vi "play-batch-raster-scan.vi"() -> ()   [LabVIEW 2017]
uses:
  raster-scan-params.ctl
  controls/PI-params.ctl
  controls/boolean_info.ctl
  controls/raster_input_meta_data.ctl
  <vilib>/userdefined/High Color/nirio_resource_hc.ctl
  controls/rasterMetaData.ctl
  <vilib>/FPGAPlugInAG/cRIO-9082/niLvFpga_Open_cRIO-9082.vi
  <vilib>/rvi/interface/common/dynamic/niFpgaDynamicAddResources.vi
  <vilib>/FPGAPlugInAG/Dynamic/niLvFpga_Reset_Dynamic.vi
  <vilib>/rvi/interface/common/niFpgaWaitOnOcc.vi
  <vilib>/Utility/error.llb/Error Cluster From Error Code.vi
  <vilib>/rvi/errors/niLvFpgaAdjustHostInterfaceError.vi
  <vilib>/FPGAPlugInAG/Dynamic/niLvFpga_Run_Dynamic.vi
  <vilib>/Utility/file.llb/Read Delimited Spreadsheet (DBL).vi
  <vilib>/FPGAPlugInAG/Dynamic/niLvFpga_Close_Dynamic.vi
  <userlib>/_matio/level5/Public/Write/Append Data Element.llb/Append Data Element (Anything).vi
  <vilib>/rvi/interface/nirviOpenFPGA/nirviOpenFPGA.xnode
  FPGA Bitfiles/afmimagingcontro_FPGATargetSPARTA_raster-scanning_DXF4O8EAjZ4.lvbitx
  <vilib>/rvi/interface/nirviMethod/nirviMethod.xnode
  <vilib>/rvi/interface/nirviReadWriteControl/nirviReadWriteControl.xnode
  <vilib>/rvi/interface/nirviCloseFPGA/nirviCloseFPGA.xnode
  <vilib>/FPGAPlugInAG/Dynamic/niLvFpga_ConfigureFifo_Dynamic.vi
  <vilib>/rvi/errors/niLvFpgaMergeErrorWithErrorCode.vi
  <vilib>/rvi/interface/Simulation/niFpgaSimulationCallBeginRW.vi
  <vilib>/FPGAPlugInAG/Dynamic/niLvFpga_ReadFifo_Dynamic.vi
  NiFpgaLv.dll
  <userlib>/_matio/level5.lvlib
  <vilib>/FPGAPlugInAG/Dynamic/niLvFpga_WriteFifo_Dynamic.vi
panel:
  out "Array 2":path[](array[path])
  out "control":dbl[](graph)
  out "error":dbl[](graph)
  out "InputMetaData":T1
  out "output-meta-data-path":path
  in  "Tab Control":enum32{"Page 1", "Debug"}(tab)
  in  "data-root":path=path "C:/Users/arnold/Documents/labview/afm_imaging/data/raster/5microns"
  in  "number-of-pixels":i32=256
  out "points_per_line":i32=250000
  out "total_num_points":i32
  in  "raise-constant (init)":sgl
  in  "raise-constant":sgl
  in  "trigger-0":bool
  in  "STOP":bool
  in  "xy-init":fxp<+/-,16,5>[](array[numeric])=[0.0, 0.0]
  in  "Ki-xy":dbl=0.01 format="%#_13g"
  out "ADC-zaxis":sgl
  out "DAC-zaxis":sgl
  in  "xy-bound":sgl=7.0
  out "current_output-data-path":path
  in  "note-blob":string
  in  "overwrite":bool
  in  "raster-scan-params":T2={"TsTicks"=1600, "Stop"=FALSE, "TOL"=0.3, "ramp-rate"=-5e-05, "z-u-max"=5.0, "PI-params"={"Ki"=0.01, "setpoint"=0.0}, "Num"=[1.0, 0.0, 0.0, 0.0, 0.0, 0.0, 0.0, 0.0, 0.0], "TF Order"=1, "Den"=[1.0, 0.0, 0.0, 0.0, 0.0, 0.0, 0.0, 0.0, 0.0]} {"ramp-rate" format="%#_5g"; "TOL" format="%#_13g"}
  in  "do-Dz":bool
  in  "do_xy_CL":bool
  out "boolean errors":T4
  in  "Z-settle-N":i16=10000
  in  "Array":string[](array[string])
  out "Actual Depth":u32
  out "Elements Remaining":u32
  out "size(s)":i32
  out "y iter":i32
  out "nsamps 2":i32
  out "Empty Elements Remaining":u32
  out "(int) y*floor(x/y)":u64
  out "elements left 2":i32=1
  out "x >= y?":bool
  out "writing stopped":bool
  out "size(s) 2":i32
  out "case-selector-feedback":i16
  out "e(0) (threshhold init)":fxp<+/-,16,5>
  out "total-time":dbl
  out "x+1":i32
  out "que timed out?":bool
  out "Error signal (previous line) 2":dbl[](graph)
  out "Waveform Graph":dbl[](graph)
  out "base y_ref (ramp)":dbl[](graph)
  out "base x_ref(triangle wave)":dbl[](graph)
  out "Intensity Graph":dbl[][](graph)
  out "Error signal (previous line)":dbl[](graph)
  # "x-axis"
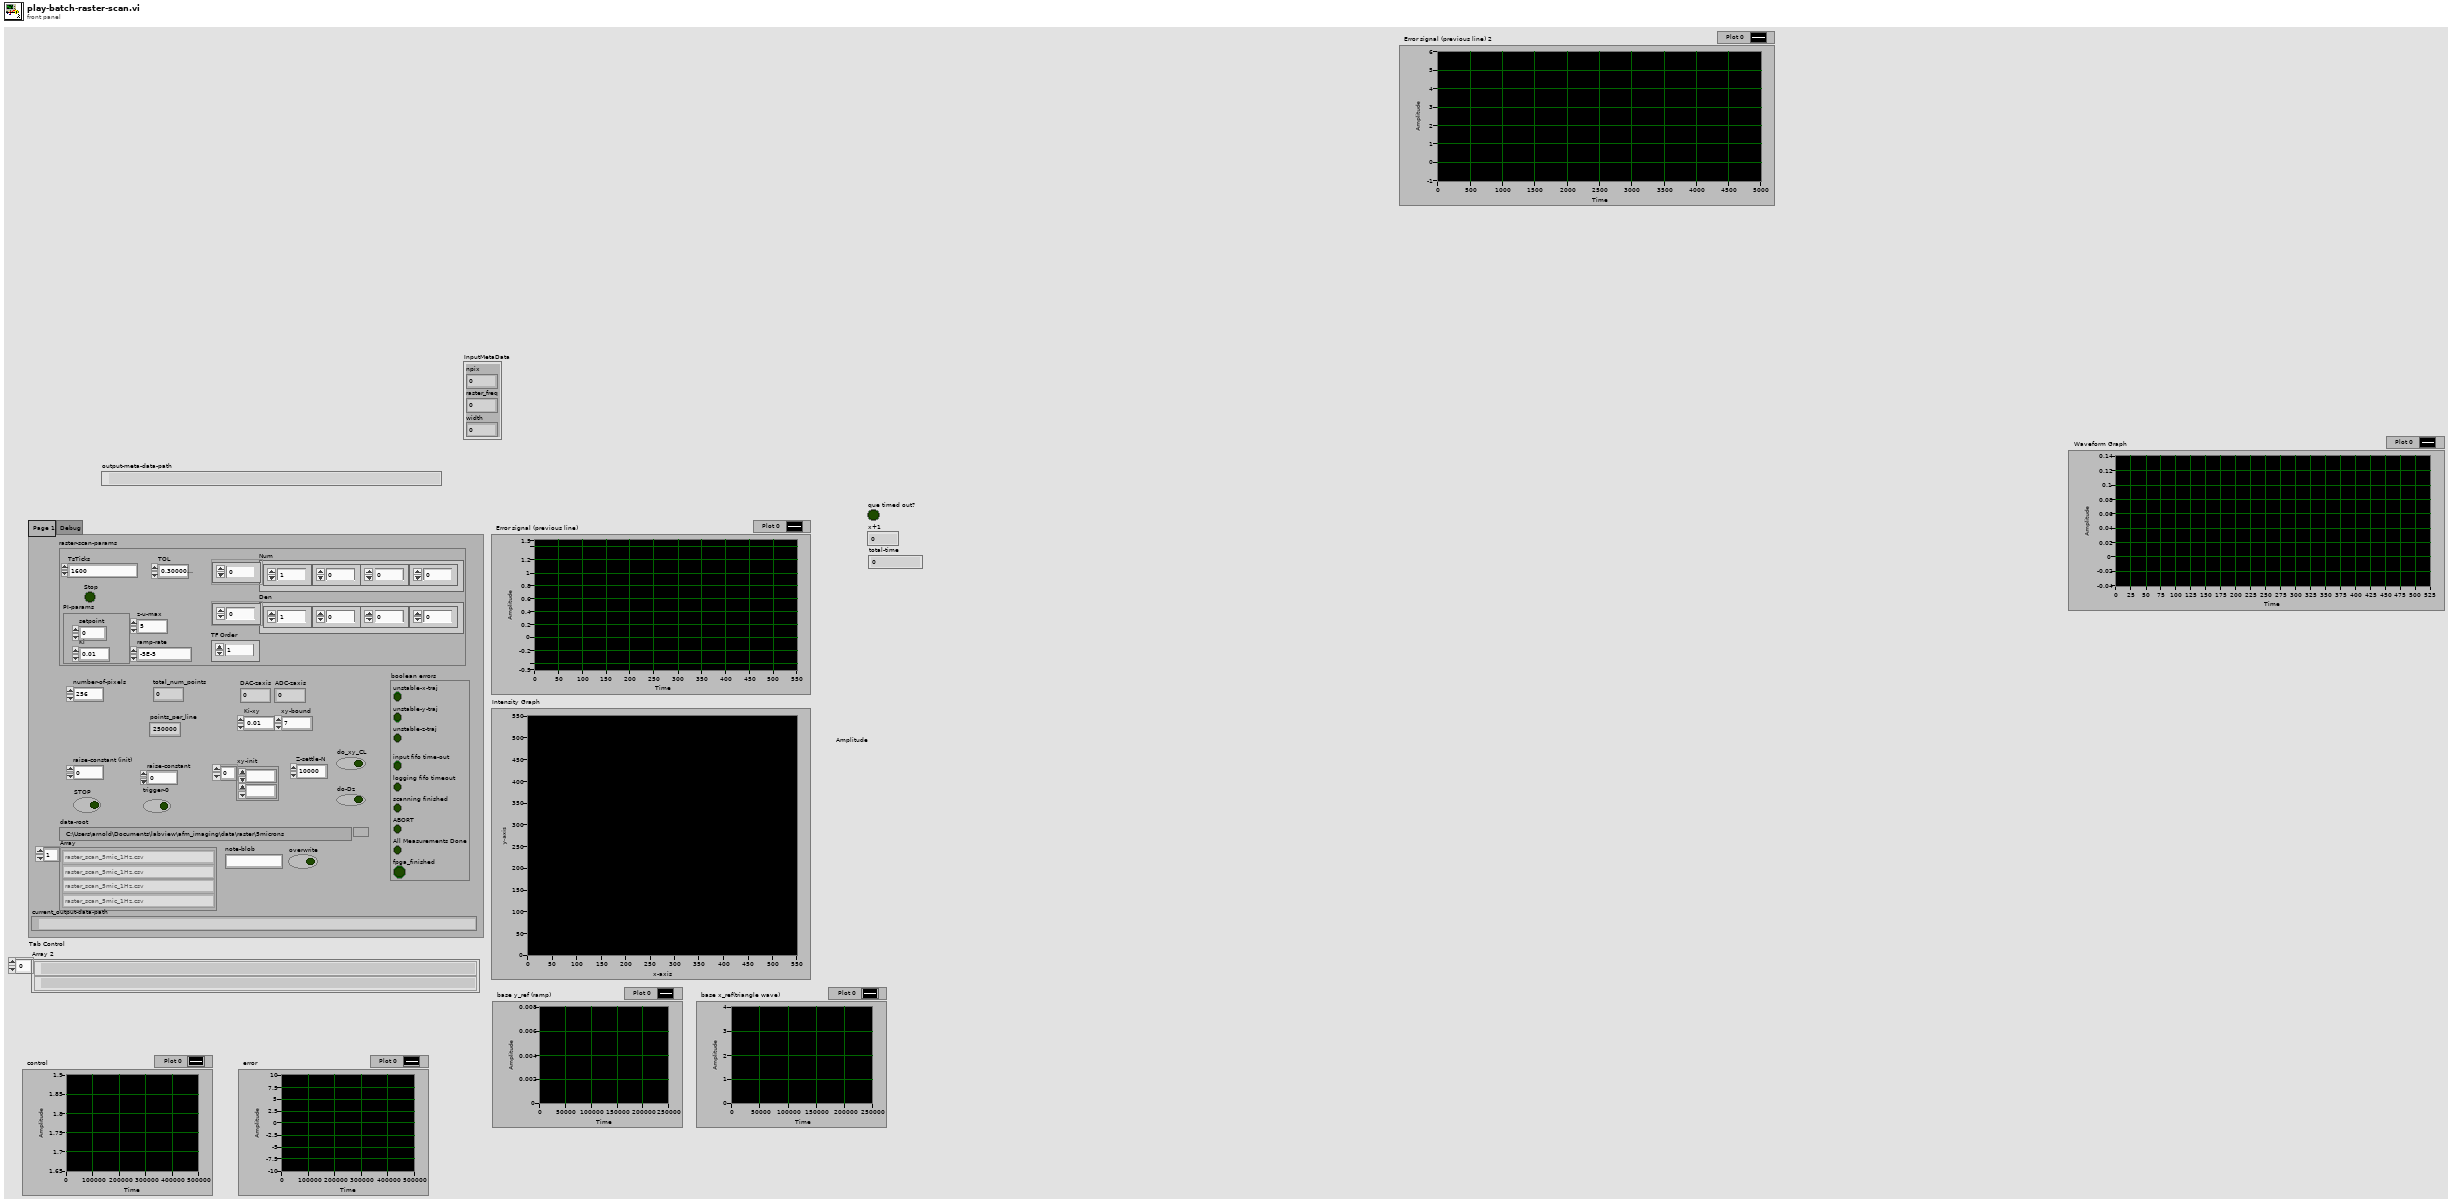
[diagram p1: front panel]
types:
  T1 = typedef "raster_input_meta_data.ctl" = cluster{"npix":dbl, "raster_freq":dbl, "width":dbl}
  T2 = typedef "raster-scan-params.ctl" = cluster{"TsTicks":u32, "Stop":bool, "TOL":sgl, "ramp-rate":sgl, "z-u-max":sgl, "PI-params":T3, "Num":sgl[], "TF Order":i32, "Den":sgl[]}
  T3 = typedef "PI-params.ctl" = cluster{"Ki":sgl, "setpoint":sgl}
  T4 = typedef "boolean_info.ctl" = cluster{"unstable-z-traj":bool, "input fifo time-out":bool, "logging fifo timeout":bool, "scanning finished":bool, "unstable-x-traj":bool, "unstable-y-traj":bool, "ABORT":bool, "All Measurements Done":bool, "fpga_finished":bool}
  T5 = typedef "nirio_resource_hc.ctl" = tag
  T6 = typedef "rasterMetaData.ctl" = cluster{"raster-scan-params":T2, "xy-bound":sgl, "DAC-zaxis":sgl, "ADC-zaxis":sgl, "Ki-xy":dbl, "total_num_points":i32, "points_per_line":i32, "number-of-lines":i32, "number-of-pixels":i32, "raster_meta_in":T1}
  T7 = enum16{"open", "replace", "create", "open or create", "replace or create", "replace or create with confirmation"}
  T8 = cluster{"unstable-z-traj":bool, "input fifo time-out":bool, "logging fifo timeout":bool, "scanning finished":bool, "unstable-x-traj":bool, "unstable-y-traj":bool, "ABORT":bool, "All Measurements Done":bool, "fpga_finished":bool}
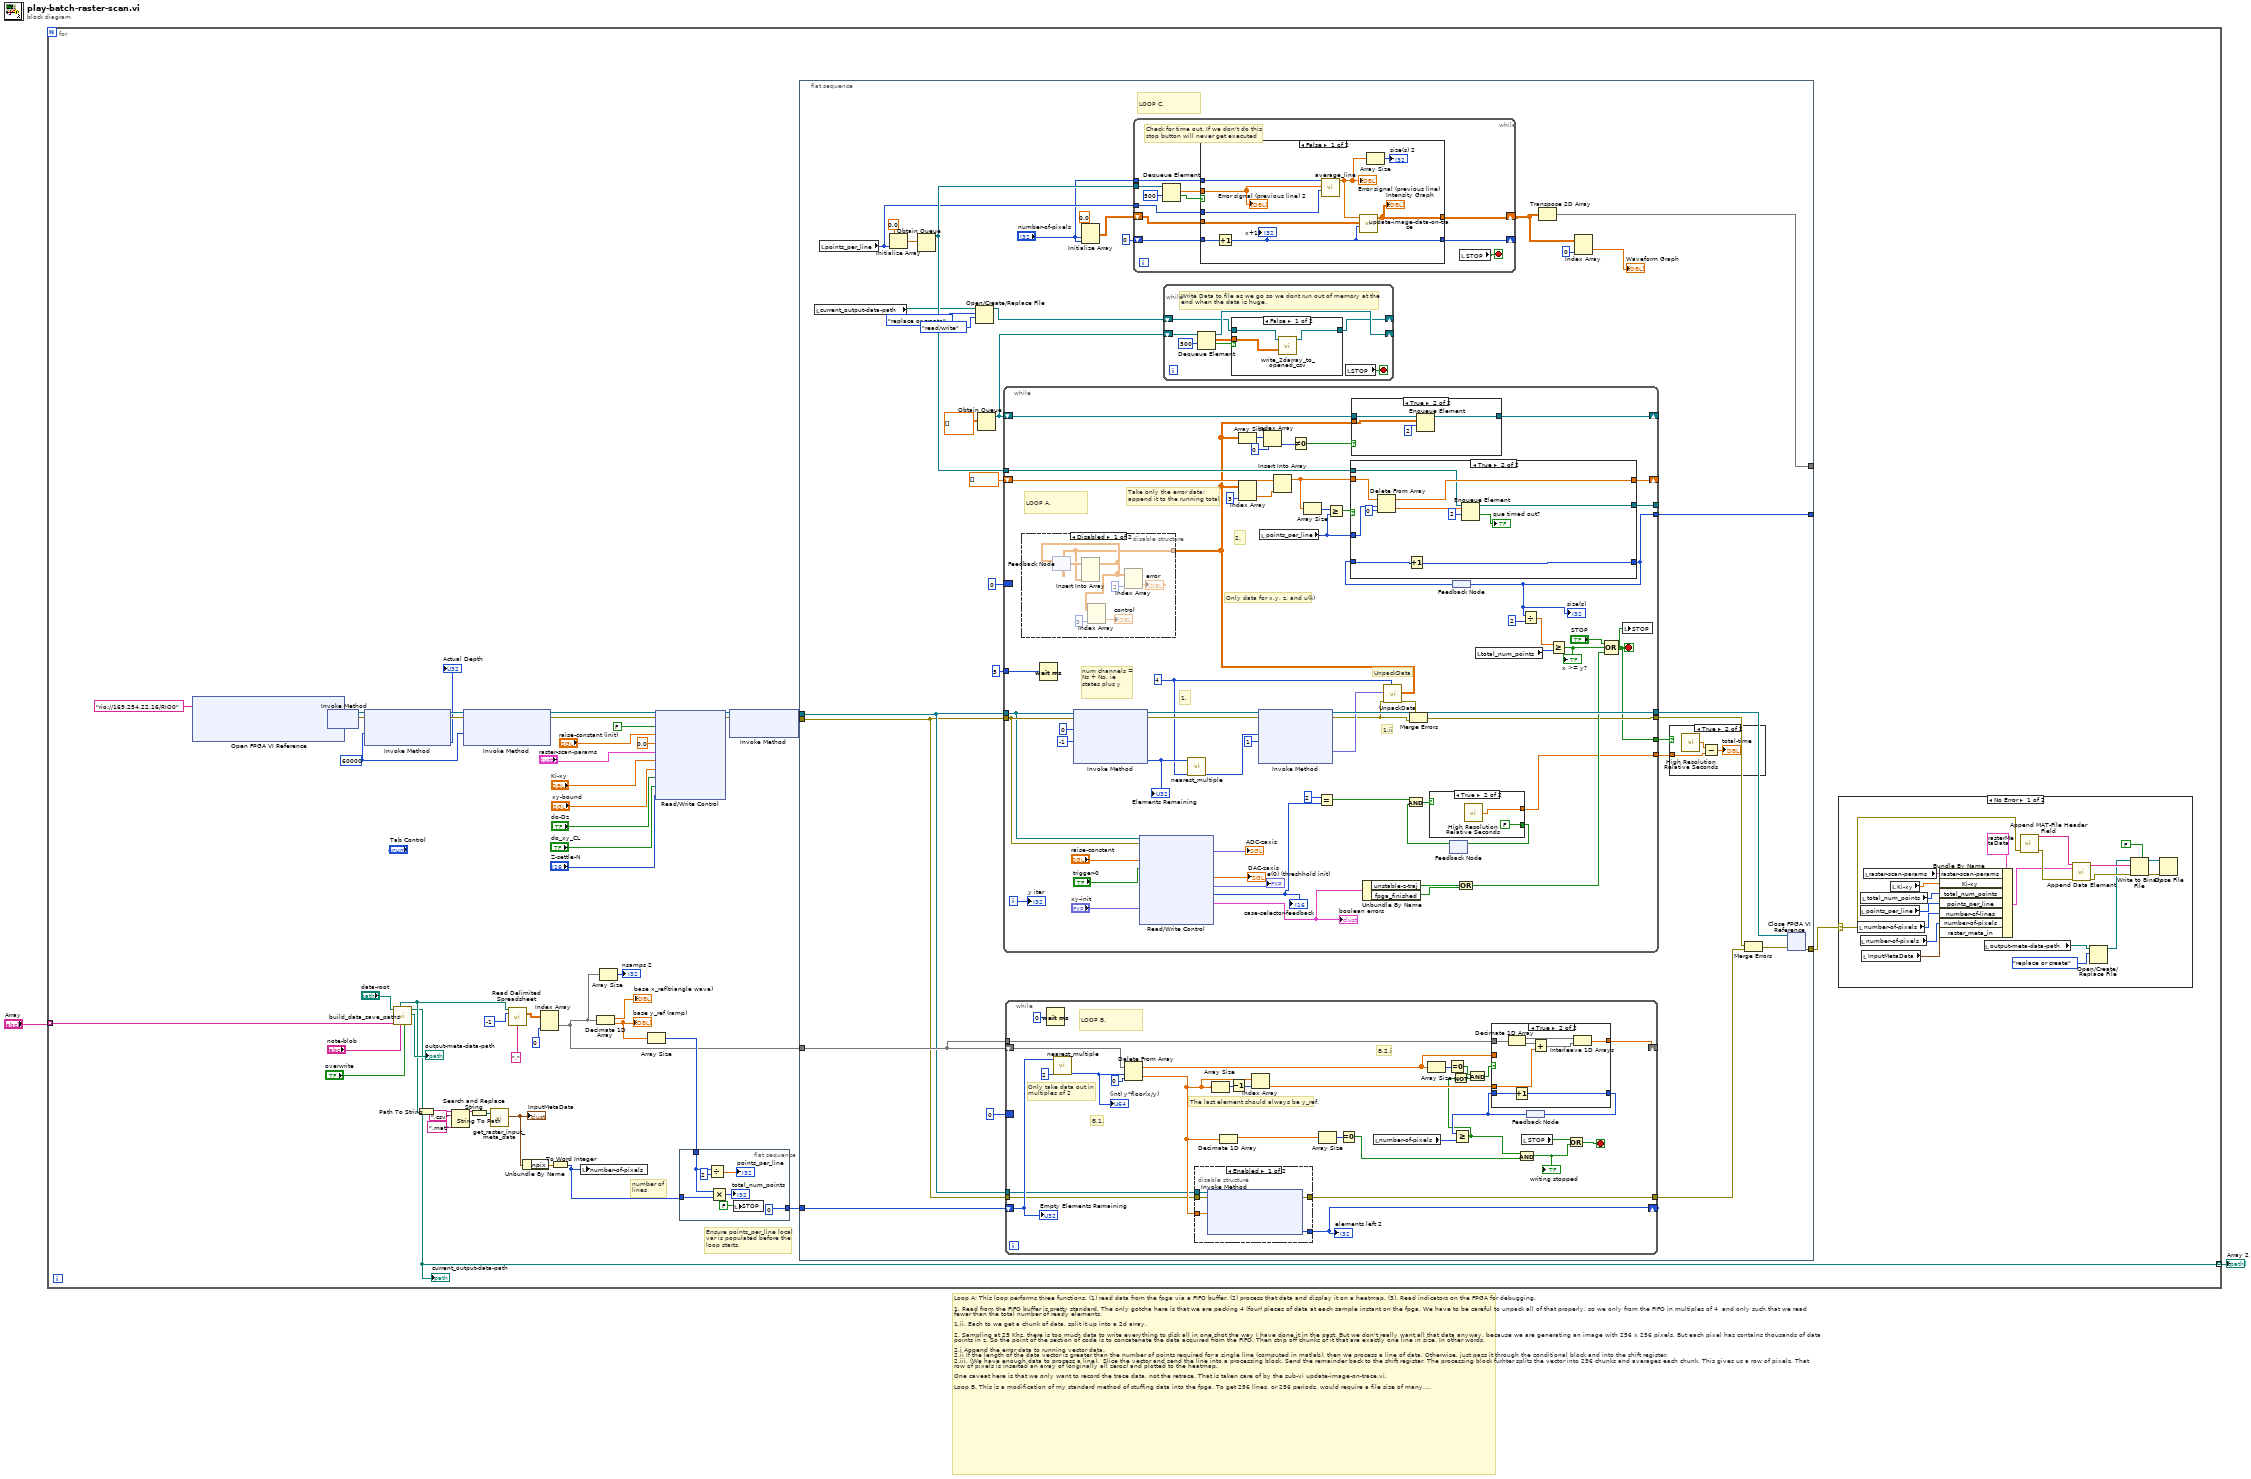
[diagram p0: block diagram]
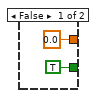
[diagram p8: hidden frame]
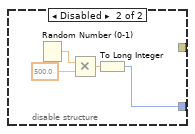
[diagram p11: hidden frame]
diagram:
  # "Loop A; This loop performs three functions. (1) read data from the fpga via a FIFO buffer. (2) process that data and display it on a heatmap. (3). Read indicators on the FPGA for debugging.\n\n1. Read from the FIFO buffer is pretty standard. The only gotcha here is that we are packing 4 (four) pieces of data at each sample instant on the fpga. We have to be careful to unpack all of that properly, so we only from the FIFO in multiples of 4  and only such that we read fewer than the total number of ready elements. \n\n1.ii. Each to we get a chunk of data, split it up into a 2d array. \n\n2. Sampling at 25 Khz, there is too much data to write everything to disk all in one shot the way I have done it in the past. But we don't really want all that data anyway, because we are generating an image with 256 x 256 pixels. But each pixel has contains thousands of data points in z. So the point of the section of code is to concatenate the data acquired from the FIFO. Then strip off chunks of it that are exactly one line in size. In other words,\n\n2.i Append the error data to running vector data.\n2.ii If the length of the data vector is greater than the number of points required for a single line (computed in matlab), then we process a line of data. Otherwise, just pass it through the conditional block and into the shift register. \n2.iii. (We have enough data to process a line).  Slice the vector and send the line into a processing block. Send the remainder back to the shift register. The processing block furhter splits the vector into 256 chunks and averages each chunk. This gives us a row of pixels. That row of pixels is inserted an array of (originally all zeros) and plotted to the heatmap.\n\nOne caveat here is that we only want to record the trace data, not the retrace. That is taken care of by the sub-vi update-image-on-trace.vi.\n\nLoop B. This is a modification of my standard method of stuffing data into the fpga. To get 256 lines, or 256 periods, would require a file size of many, many gigibtyes. SO the point here is to only use a single period of the triangle wave and corresponding ramp signal. Everytime we exauhst that data, re-cycle the same data and keep pumping it back in. The one tricky part here is that we have to be careful to shift the original ramp data up by the appropriate amount. We also have to take special care because of how the data is packed from matlab. [x(1), y(1), x(2), y(2)...].\n\nThe first iteration of the loop, we don't push any data in. All we do is get the number of empty elements.\n\nB.1 Each iteration, strip off ' empty elements ' elements from the array and send them to FIFO. \nB.2.i Is the remaining array empty?\nB.2.ii Grab the very last element. We need this"
  n1 = for {
    tunnel: "Array" -> [w4] mode=indexing
    tunnel: [w3] -> w1 mode=indexing
    w50 = 60000
    # "number of \nlines"
    # "Ensure points_per_line local\nvar is populated before the\nloop starts."
    n2 = xnode "Open FPGA VI Reference"("resource name"=T5 "rio://169.254.22.16/RIO0") -> ("FPGA VI Reference Out"=w49:refnum<k20>, "error out"=w48:errorcluster)  [unwired: 1 in]
    n3 = xnode "Invoke Method"("FPGA VI Reference In"=w49, "error in"=w48) -> ("FPGA VI Reference Out"=w44:refnum<k20>, "error out"=w43:errorcluster)
    n4 = xnode "Invoke Method"("FPGA VI Reference In"=w44, "error in"=w43, "Requested Depth"=w50) -> ("FPGA VI Reference Out"=w45:refnum<k20>, "error out"=w46:errorcluster, "Actual Depth"=→"Actual Depth":u32)
    n5 = call "build_data_save_paths.vi"("overwrite"="overwrite", "note-blob"="note-blob", "base-file-name"=w4, "data-root"="data-root") -> ("output-meta-data-path"=→"output-meta-data-path":path, "output-data-path"=w3:path, "input-data-path"=w13:path)  [unwired: 3 in, 2 out]
    "current_output-data-path" <- w3
    n6 = Path To String(path=w13) -> (string=w12:string)
    n7 = Search and Replace String(input string=w12, search string=".csv", replace string=".mat" ("replace string (\"\")")) -> (result string=w9:string)  [unwired: 5 in, 3 out]
    n8 = xnode "Invoke Method"("FPGA VI Reference In"=w45, "error in"=w46, "Requested Depth"=w50) -> ("FPGA VI Reference Out"=w52:refnum<k20>, "error out"=w51:errorcluster)  [unwired: 1 out]
    n9 = String To Path(string=w9) -> (path=w8:path)
    n10 = call "get_raster_input_meta_data.vi"("Path"=w8) -> ("cluster"=w7:T1)  [unwired: 10 in]
    "InputMetaData" <- w7
    n11 = call-poly <vilib>:"Read Delimited Spreadsheet.vi"("file path (dialog if empty)"=w13, "number of rows (all:-1)"=-1, "delimiter (\\t)"=",") -> ("all rows"=w30:dbl[][])  [unwired: 7 in, 5 out]
    n12 = Unbundle By Name(w7) -> ("npix"=w6:dbl)
    n13 = Index Array(array=w30, index (col)=0 ("dimension size")) -> (element=w29:dbl[])  [unwired: 1 in]
    n14 = To Word Integer(number=w6) -> (16bit integer=w5:i16)
    n15 = local write "number-of-pixels"(w5) -> ()
    n16 = Decimate 1D Array(w29) -> (→"base x_ref(triangle wave)":dbl[], w36:dbl[])
    "base y_ref (ramp)" <- w36
    n17 = Array Size(array=w29) -> (size(s)=→"nsamps 2":i32)
    n18 = Array Size(array=w36) -> (size(s)=w34:i32)
    n19 = xnode "Read/Write Control"("FPGA VI Reference In"=w52, "error in"=w51, "trigger-0"=FALSE ("constant 2 lower"), "raise-constant"="raise-constant (init)", "u(0)"=sgl 0.0, "raster-scan-params"="raster-scan-params", "Ki-xy"="Ki-xy", "xy-bound"="xy-bound", "do-Dz"="do-Dz", "do_xy_CL"="do_xy_CL", "Z-settle-N"="Z-settle-N") -> ("FPGA VI Reference Out"=w26:refnum<k20>, "error out"=w25:errorcluster)
    n20 = flat-sequence {
      tunnel: [0] -> w35
      tunnel: w34 -> [w285]
      tunnel: w5 -> [w288]
      frame #0 {
        n21 = Divide(x=w285, y=2) -> (x/y=→"points_per_line":dbl)
        n22 = Multiply(x=w285, y=w288) -> (x*y=→"total_num_points":i32)
        n23 = local write "STOP"(FALSE ("STOP")) -> ()
      }
    }
    n24 = xnode "Invoke Method"("FPGA VI Reference In"=w26, "error in"=w25) -> ("FPGA VI Reference Out"=w23:refnum<k20>, "error out"=w24:errorcluster)  [unwired: 1 in]
    n25 = flat-sequence {
      tunnel: [w82] -> _
      tunnel: w23 -> [w91]
      tunnel: w24 -> [w90]
      tunnel: w35 -> [w103]
      tunnel: w29 -> [w92]
      tunnel: [w76] -> _
      tunnel: [w73] -> w17
      frame #0 {
        # "LOOP C."
        n26 = local read "current_output-data-path"() -> (w75:path)
        n27 = local read "points_per_line"() -> (w88:i32)
        n28 = Initialize Array(0.0 ("element"), w88) -> (w97:dbl[])
        n29 = Obtain Queue(element data type=w97) -> (queue out=w94:refnum<queue>)  [unwired: 4 in, 2 out]
        n30 = Open/Create/Replace File(file path (use dialog)=w75, operation (0:open)=T7."replace or create", access (0:read/write)=enum16{"read/write", "read-only", "write-only"}."read/write") -> (refnum out=w77:refnum<file>)  [unwired: 3 in, 2 out]
        n31 = Obtain Queue(element data type=dbl[][] []) -> (queue out=w80:refnum<queue>)  [unwired: 4 in, 2 out]
        n32 = while {
          tunnel: 5 -> [w202]
          tunnel: w91 -> [w193]
          tunnel: w90 -> [w194]
          tunnel: [w173] -> w85
          tunnel: [w196] -> w86
          shift-right: [w185] -> _
          shift-left: dbl[] [] -> [w183]
          border: 0 ("disabled index (col)") -> [_]
          tunnel: w94 -> [w164]
          tunnel: [w163] -> _
          tunnel: [w161] -> w84
          tunnel: [w154] -> w83
          shift-right: [w148] -> _
          shift-left: w80 -> [w147]
          tunnel: [w146] -> w76
          i -> [w192]
          stop <- w161 stop-if-true
          w170 = u32 4 ("y")
          # "2."
          # "1.ii"
          # "1."
          # "LOOP A."
          # "Take only the error data;\nappend it to the running total"
          # "num channels = Ns + No, ie states plus y"
          # "Only data for x,y, z, and u(k)"
          # "UnpackData"
          n33 = Wait (ms)(milliseconds to wait=w202) -> ()  [unwired: 1 out]
          n34 = xnode "Invoke Method"("FPGA VI Reference In"=w193, "error in"=w194, "Number of Elements"=0 ("Timeout (ms)"), "Timeout (ms)"=-1) -> ("FPGA VI Reference Out"=w198:refnum<k20>, "error out"=w199:errorcluster, "Elements Remaining"=w171:u32)  [unwired: 1 out]
          "Elements Remaining" <- w171
          n35 = xnode "Read/Write Control"("FPGA VI Reference In"=w193, "error in"=w194, "raise-constant"="raise-constant", "trigger-0"="trigger-0", "xy-init"="xy-init") -> ("ADC-zaxis"=→"ADC-zaxis":fxp<+/-,24,5>, "DAC-zaxis"=→"DAC-zaxis":sgl, "e(0) (threshhold init)"=→"e(0) (threshhold init)":fxp<+/-,16,5>, "current-case"=w160:i16, "boolean errors"=w145:T8)  [unwired: 1 in, 2 out]
          "case-selector-feedback" <- w160
          "boolean errors" <- w145
          n36 = call "nearest_multiple.vi"("numChan"=w170, "N"=w171) -> ("(int) y*floor(x/y)"=w169:u64)  [unwired: 9 in]
          n37 = xnode "Invoke Method"("FPGA VI Reference In"=w198, "error in"=w199, "Number of Elements"=w169, "Timeout (ms)"=1) -> ("FPGA VI Reference Out"=w196:refnum<k20>, "error out"=w175:errorcluster, "Data"=w195:fxp<+/-,16,5>[])  [unwired: 1 out]
          n38 = local read "points_per_line"() -> (w172:i32)
          n39 = Equal?(x=i16 2, y=w160) -> (x = y?=w158:bool)
          n40 = Unbundle By Name(w145) -> ("unstable-z-traj"=w166:bool, "fpga_finished"=w165:bool)
          n41 = call "UnpackData.vi"("NumChannels"=w170, "error In"=w175, "1D Data In"=w195) -> ("error Out"=w174:errorcluster, "2D Data Out"=w144:dbl[][])  [unwired: 7 in]
          n42 = disable-structure shown="Disabled" {
            disable-tunnel: w144 -> [w203 _]
            frame Disabled {
              n43 = feedback #1(w203) -> (w209:dbl[][])
              n44 = Insert Into Array(array=w209, new element=w203) -> (w204:dbl[][])  [unwired: 2 in]
              n45 = feedback-in #1(w204) -> ()
              n46 = Index Array(array=w204, index (col)=3 ("disabled index (col)")) -> (element=→"control":dbl[])  [unwired: 1 in]
              n47 = Index Array(array=w204, index (col)=2 ("disabled index (col)")) -> (element=→"error":dbl[])  [unwired: 1 in]
            }
            frame Enabled {
            }
          }
          n48 = Array Size(array=w144) -> (size(s)=w152:i32[])
          n49 = Index Array(array=w144, index (col)=3 ("disabled index (col)")) -> (element=w182:dbl[])  [unwired: 1 in]
          n50 = Index Array(array=w152, index=0) -> (element=w150:i32)
          n51 = Insert Into Array(array=w183, new element=w182) -> (w153:dbl[])  [unwired: 1 in]
          n52 = Not Equal To 0?(x=w150) -> (x != 0?=w149:bool)
          n53 = Array Size(array=w153) -> (size(s)=w184:i32)
          n54 = Greater Or Equal?(x=w184, y=w172) -> (x >= y?=w181:bool)
          n55 = case shown="True" w149 {
            tunnel: w147 -> [w210 w214]
            tunnel: w144 -> [_ w212]
            tunnel: [w210 w211] -> w148
            frame False {
            }
            frame True {
              n56 = Enqueue Element(queue=w214, element=w212, timeout in ms (-1)=2) -> (queue out=w211:refnum<queue>)  [unwired: 1 in, 2 out]
            }
          }
          n57 = Merge Errors(w174, w175) -> (w173:errorcluster)
          n58 = feedback #2() -> (w156:bool)  [unwired: 1 in]
          n59 = And(x=w158, y=w156) -> (x .and. y?=w159:bool)
          n60 = case shown="True" w159 {
            tunnel: [TRUE FALSE] -> w157
            tunnel: [0.0 ("relative seconds") w217] -> w154
            frame False {
            }
            frame True {
              n61 = call <vilib>:"High Resolution Relative Seconds.vi"() -> ("relative seconds"=w217:dbl)
            }
          }
          n62 = feedback-in #2(w157) -> ()
          n63 = feedback #3() -> (w180:i32)
          n64 = case shown="True" w181 {
            tunnel: [w221 w230] -> w185
            tunnel: w153 -> [w221 w232]
            tunnel: w180 -> [w220 w229]
            tunnel: [w220 w228] -> w146
            tunnel: w172 -> [_ w227]
            tunnel: w164 -> [w219 w225]
            tunnel: [w219 w224] -> w163
            frame False {
            }
            frame True {
              n65 = Delete From Array(array=w232, length=w227, index=0) -> (deleted portion=w226:dbl[], array with subset deleted=w230:dbl[])
              n66 = Increment(x=w229) -> (x+1=w228:i32)
              n67 = Enqueue Element(queue=w225, element=w226, timeout in ms (-1)=2) -> (queue out=w224:refnum<queue>, timed out?=→"que timed out?":bool)  [unwired: 1 in, 1 out]
            }
          }
          "size(s)" <- w146
          n68 = feedback-in #3(w146) -> ()
          n69 = Or(x=w166, y=w165) -> (x .or. y?=w176:bool)
          n70 = local read "total_num_points"() -> (w179:i32)
          n71 = Divide(x=w146, y=2) -> (x/y=w168:dbl)
          n72 = Greater Or Equal?(x=w168, y=w179) -> (x >= y?=w177:bool)
          "x >= y?" <- w177
          n73 = Compound Arithmetic op=OR("STOP", w177, w176) -> (w161:bool)
          n74 = local write "STOP"(w161) -> ()
          "y iter" <- w192
        }
        n75 = while {
          shift-right: [w262] -> _
          shift-left: w103 -> [w257]
          shift-right: [w250] -> _
          shift-left: w92 -> [w263]
          tunnel: w92 -> [w248]
          tunnel: [w254] -> w104
          tunnel: w91 -> [w246]
          tunnel: w90 -> [w245]
          border: 0 ("Timeout (ms)") -> [_]
          stop <- w258 stop-if-true
          # "B.2.i"
          # "B.1."
          # "LOOP B."
          # "Only take data out in \nmultiples of 2"
          # "The last element should always be y_ref."
          n76 = Wait (ms)(milliseconds to wait=0) -> ()  [unwired: 1 out]
          n77 = call "nearest_multiple.vi"("numChan"=u32 2 ("Empty Elements Remaining"), "N"=w257) -> ("(int) y*floor(x/y)"=w256:u64)  [unwired: 9 in]
          "(int) y*floor(x/y)" <- w256
          n78 = Delete From Array(array=w263, length=w256, index=0) -> (deleted portion=w251:dbl[], array with subset deleted=w249:dbl[])
          n79 = disable-structure shown="Enabled" {
            disable-tunnel: [w278 w279] -> w262
            disable-tunnel: w251 -> [w277 _]
            disable-tunnel: [w276 _] -> w254
            disable-tunnel: w246 -> [w275 _]
            disable-tunnel: w245 -> [w274 _]
            frame Enabled {
              n80 = xnode "Invoke Method"("FPGA VI Reference In"=w275, "error in"=w274, "Data"=w277) -> ("error out"=w276:errorcluster, "Empty Elements Remaining"=w278:u32)  [unwired: 1 in, 1 out]
            }
            frame Disabled {
              n81 = Random Number (0-1)() -> (number: 0 to 1=w282:dbl)
              n82 = Multiply(x=w282, y=500.0) -> (x*y=w280:dbl)
              n83 = To Long Integer(number=w280) -> (32bit integer=w279:i32)
            }
          }
          "elements left 2" <- w262
          n84 = Array Size(array=w251) -> (size(s)=w252:i32)
          n85 = Decimate 1D Array(w251) -> (w237:dbl[])  [unwired: 1 out]
          n86 = Decrement(x=w252) -> (x-1=w253:i32)
          n87 = Index Array(array=w251, index=w253) -> (element=w247:dbl)
          n88 = Array Size(array=w237) -> (size(s)=w239:i32)
          n89 = Equal To 0?(x=w239) -> (x = 0?=w238:bool)
          n90 = local read "number-of-pixels"() -> (w243:i32)
          n91 = Array Size(array=w249) -> (size(s)=w260:i32)
          n92 = Equal To 0?(x=w260) -> (x = 0?=w236:bool)
          n93 = local read "STOP"() -> (w259:bool)
          n94 = feedback #4() -> (w241:i32)
          n95 = Greater Or Equal?(x=w241, y=w243) -> (x >= y?=w234:bool)
          n96 = Not(x=w234) -> (.not. x?=w235:bool)
          n97 = And(x=w236, y=w235) -> (x .and. y?=w233:bool)
          n98 = case shown="True" w233 {
            tunnel: [w265 w268] -> w250
            tunnel: w249 -> [w265 _]
            tunnel: w248 -> [_ w273]
            tunnel: w247 -> [_ w271]
            tunnel: [w264 w267] -> w242
            tunnel: w241 -> [w264 w266]
            frame False {
            }
            frame True {
              n99 = Decimate 1D Array(w273) -> (w270:dbl[], w272:dbl[])
              n100 = Increment(x=w266) -> (x+1=w267:i32)
              n101 = Add(x=w272, y=w271) -> (x+y=w269:dbl[])
              n102 = Interleave 1D Arrays(w270, w269) -> (w268:dbl[])
            }
          }
          n103 = And(x=w234, y=w238) -> (x .and. y?=w240:bool)
          "writing stopped" <- w240
          n104 = feedback-in #4(w242) -> ()
          n105 = Or(x=w259, y=w240) -> (x .or. y?=w258:bool)
          "Empty Elements Remaining" <- w257
        }
        n106 = Initialize Array(0.0 ("element"), "number-of-pixels", "number-of-pixels") -> (w96:dbl[][])
        n107 = while {
          shift-right: [w132] -> w93
          shift-left: w96 -> [w131]
          shift-right: [w129] -> _
          shift-left: 0 ("disabled index (col)") -> [w130]
          tunnel: w88 -> [w128]
          tunnel: w94 -> [w127]
          tunnel: "number-of-pixels" -> [w122]
          stop <- w125 stop-if-true
          # "Check for time out. If we don't do this\nstop button will never get executed"
          n108 = Dequeue Element(queue=w127, timeout in ms (-1)=500) -> (element=w126:dbl[], timed out?=w123:bool)  [unwired: 1 in, 2 out]
          n109 = case shown="False" w123 {
            tunnel: [w141 w142] -> w132
            tunnel: w131 -> [w140 w142]
            tunnel: w130 -> [w139 w143]
            tunnel: [w138 w143] -> w129
            tunnel: w128 -> [w137 _]
            tunnel: w126 -> [w136 _]
            tunnel: w122 -> [w133 _]
            frame False {
              n110 = Increment(x=w139) -> (x+1=w138:i32)
              "x+1" <- w138
              n111 = call "average_line.vi"("data-pts-per-line"=w137, "raw-data-row"=w136, "number-of-pixels"=w133) -> ("avg-data-row"=w135:dbl[])  [unwired: 8 in]
              "Error signal (previous line)" <- w135
              n112 = call "update-image-data-on-trace.vi"("iterator"=w138, "master-image-data-n"=w140, "avg-data-row"=w135) -> ("master-image-data-out"=w141:dbl[][])  [unwired: 8 in]
              "Intensity Graph" <- w141
              n113 = Array Size(array=w135) -> (size(s)=→"size(s) 2":i32)
              "Error signal (previous line) 2" <- w136
            }
            frame True {
            }
          }
          n114 = local read "STOP"() -> (w125:bool)
        }
        n115 = while {
          shift-right: [w109] -> _
          shift-left: w80 -> [w110]
          shift-right: [w107] -> _
          shift-left: w77 -> [w108]
          stop <- w112 stop-if-true
          # "Write Data to file as we go so we dont run out of memory at the \nend when the data is huge."
          n116 = Dequeue Element(queue=w110, timeout in ms (-1)=500) -> (queue out=w109:refnum<queue>, element=w111:dbl[][], timed out?=w113:bool)  [unwired: 1 in, 1 out]
          n117 = case shown="False" w113 {
            tunnel: w111 -> [w115 _]
            tunnel: w108 -> [w117 w118]
            tunnel: [w116 w118] -> w107
            frame False {
              n118 = call "write_2darray_to_opened_csv.vi"("Data_in"=w115, "file_ref_in"=w117) -> ("file_ref_out"=w116:refnum<file>)  [unwired: 9 in]
            }
            frame True {
            }
          }
          n119 = local read "STOP"() -> (w112:bool)
        }
        n120 = Transpose 2D Array(2D array=w93) -> (transposed array=w82:dbl[][])
        n121 = Index Array(array=w93, index (col)=0 ("disabled index (col)")) -> (element=→"Waveform Graph":dbl[])  [unwired: 1 in]
        n122 = case shown="True" w84 {
          tunnel: w83 -> [_ w121]
          frame False {
          }
          frame True {
            n123 = call <vilib>:"High Resolution Relative Seconds.vi"() -> ("relative seconds"=w120:dbl)
            n124 = Subtract(x=w120, y=w121) -> (x-y=→"total-time":dbl)
          }
        }
        n125 = Merge Errors(w85, w104) -> (w74:errorcluster)
        n126 = xnode "Close FPGA VI Reference"("FPGA VI Reference In"=w86, "error in"=w74) -> ("error out"=w73:errorcluster)
      }
    }
    n127 = case shown="No Error" w17 {
      selector: w17 -> [w61 _]
      frame No Error {
        n128 = local read "number-of-pixels"() -> (w55:i32)
        n129 = local read "points_per_line"() -> (w56:i32)
        n130 = local read "number-of-pixels"() -> (w54:i32)
        n131 = local read "total_num_points"() -> (w57:i32)
        n132 = local read "InputMetaData"() -> (w53:T1)
        n133 = local read "raster-scan-params"() -> (w59:T2)
        n134 = local read "Ki-xy"() -> (w58:dbl)
        n135 = Bundle By Name(cluster=T6 {"raster-scan-params"={"TsTicks"=1600, "Stop"=TRUE, "TOL"=0.3, "ramp-rate"=-5e-05, "z-u-max"=5.0, "PI-params"={"Ki"=0.01, "setpoint"=0.0}, "Num"=[1.0, 0.0, 0.0, 0.0, 0.0, 0.0, 0.0, 0.0, 0.0], "TF Order"=3, "Den"=[1.0, 0.0, 0.0, 0.0, 0.0, 0.0, 0.0, 0.0, 0.0]}, "xy-bound"=7.0, "DAC-zaxis"=0.0, "ADC-zaxis"=0.0, "Ki-xy"=0.01, "total_num_points"=0, "points_per_line"=250000, "number-of-lines"=256, "number-of-pixels"=256, "raster_meta_in"={"npix"=0.0, "raster_freq"=0.0, "width"=0.0}} ("Cluster"), "raster-scan-params"=w59, "Ki-xy"=w58, "total_num_points"=w57, "points_per_line"=w56, "number-of-lines"=w55, "number-of-pixels"=w54, "raster_meta_in"=w53) -> (w60:T6)
        n136 = local read "output-meta-data-path"() -> (w63:path)
        n137 = call <userlib>:"Append MAT-File Header Field.vi"("error"=w61) -> ("result string"=w72:string, "error out"=w66:errorcluster)  [unwired: 13 in]
        n138 = call-poly <userlib>:"Append Data Element.vi"("initial string"=w72, "data"=w60, "error in (no error)"=w66) -> ("result string"=w70:string, "error out"=w71:errorcluster)  [unwired: 11 in]
        n139 = Open/Create/Replace File(file path (use dialog)=w63, operation (0:open)=T7."replace or create") -> (refnum out=w65:refnum<file>)  [unwired: 4 in, 2 out]
        n140 = Write to Binary File(file (use dialog)=w65, data=w70, error in=w71, 5:FALSE ("prepend array or string size? (T)")) -> (refnum out=w67:refnum<file>, error out=w68:errorcluster)  [unwired: 2 in, 1 out]
        n141 = Close File(refnum=w67, error in=w68) -> ()  [unwired: 2 out]
      }
      frame Error {
      }
    }
  }
  "Array 2" <- w1
